vi "Open Server VI ref.vi"(8 "error in (no error)":errorcluster) -> (0 "error out":errorcluster, 3 "VI out":T1)   [LabVIEW 2018]
doc: "Author: Scott Hannahs <sth@magnet.fsu.edu>\nCopyright 2018 Florida State University, All rights reserved."
uses:
  Net Conn Handler VI.ctl
  <vilib>/Utility/error.llb/DialogType.ctl
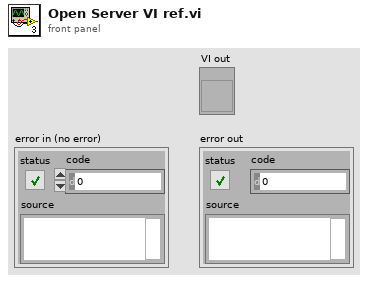
[diagram p1: front panel]
types:
  T1 = typedef "Net Conn Handler VI.ctl" = refnum<vi>
  T2 = typedef "DialogType.ctl" = u16
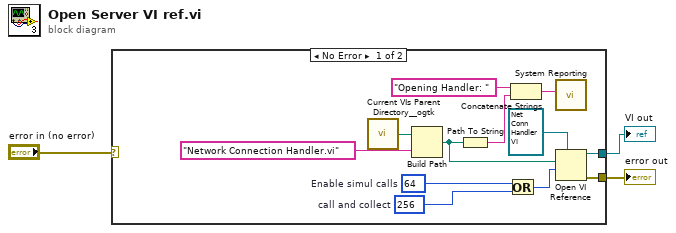
[diagram p0: block diagram]
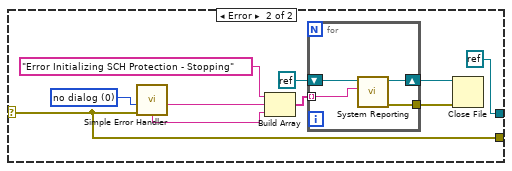
[diagram p2: hidden frame]
diagram:
  n1 = case shown="No Error" "error in (no error)" {
    selector: "error in (no error)" -> [_ w24]
    tunnel: [w6 w24] -> w3
    tunnel: [w7 refnum<k0> refnum] -> w2
    frame No Error {
      w13 = 256  # call and collect
      w15 = 64  # Enable simul calls
      n2 = call <userlib>:"Current VIs Parent Directory__ogtk.vi"() -> ("Parent Directory (+ Relative)"=w5:path)  [unwired: 5 in]
      n3 = Build Path(base path=w5, name or relative path="Network Connection Handler.vi") -> (appended path=w10:path)
      n4 = Path To String(path=w10) -> (string=w11:string)
      n5 = Or(x=w15, y=w13) -> (x .or. y?=w14:i32)
      n6 = Concatenate Strings("Opening Handler: " ("string"), w11) -> (w8:string)
      n7 = call "System Reporting.vi"("String"=w8) -> ()  [unwired: 9 in, 2 out]
      n8 = Open VI Reference(type specifier VI Refnum (for type only)=T1 refnum ("Handler VI ref"), vi path=w10, options=w14) -> (vi reference=w7:T1, error out=w6:errorcluster)  [unwired: 3 in]
    }
    frame Error {
      w21 = T2 0 items=["no dialog", "OK message", "continue or stop message", "OK message + warnings", "continue/stop + warnings"] ("type of dialog (OK msg:1)")
      n9 = call <vilib>:"Simple Error Handler.vi"("type of dialog (OK msg:1)"=w21, "error in (no error)"=w24) -> ("source out"=w23:string, "message"=w22:string)  [unwired: 3 in, 3 out]
      n10 = Build Array("Error Initializing SCH Protection - Stopping" ("text"), w23, w22) -> (w18:string[])
      n11 = for {
        tunnel: [w29] -> w20
        tunnel: w18 -> [w27] mode=indexing
        shift-right: [w28] -> w19
        shift-left: refnum<k0> refnum ("Byte Stream File out") -> [w26]
        n12 = call "System Reporting.vi"("String"=w27, "Byte Stream File in"=w26) -> ("Error Out"=w29:errorcluster, "Byte Stream File out"=w28:refnum<file>)  [unwired: 8 in]
      }
      n13 = Close File(refnum=w19, error in=w20) -> ()  [unwired: 2 out]
    }
  }
  "error out" <- w3
  "VI out" <- w2
